vi "Run Test Suite.vi"() -> ()   [LabVIEW 2013]
uses:
  <vilib>/addons/_JKI Toolkits/Caraya/classes/Test/Test.lvclass
panel:
  out "error out":errorcluster
  # "Run Me"
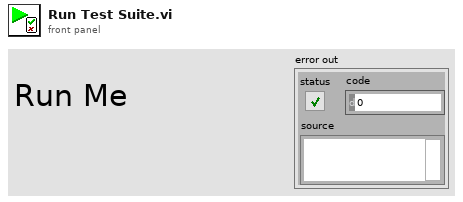
[diagram p1: front panel]
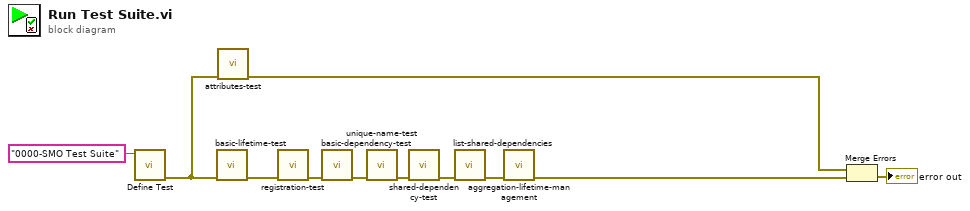
[diagram p0: block diagram]
diagram:
  n1 = call <vilib>:"Define Test.vi"("Label (VI Title)"="0000-SMO Test Suite") -> ("error out"=w1:errorcluster)  [unwired: 10 in]
  n2 = call "basic-lifetime-test.vi"("error in (no error)"=w1) -> ("error out"=w9:errorcluster)  [unwired: 10 in]
  n3 = call "attributes-test.vi"("error in (no error)"=w1) -> ("error out"=w2:errorcluster)  [unwired: 10 in]
  n4 = call "registration-test.vi"("error in (no error)"=w9) -> ("error out"=w8:errorcluster)  [unwired: 10 in]
  n5 = call "basic-dependency-test.vi"("error in (no error)"=w8) -> ("error out"=w10:errorcluster)  [unwired: 10 in]
  n6 = call "unique-name-test.vi"("error in (no error)"=w10) -> ("error out"=w7:errorcluster)  [unwired: 10 in]
  n7 = call "shared-dependency-test.vi"("error in (no error)"=w7) -> ("error out"=w6:errorcluster)  [unwired: 10 in]
  n8 = call "list-shared-dependencies.vi"("error in (no error)"=w6) -> ("error out"=w5:errorcluster)  [unwired: 10 in]
  n9 = call "aggregation-lifetime-management.vi"("error in (no error)"=w5) -> ("error out"=w4:errorcluster)  [unwired: 10 in]
  n10 = Merge Errors(w2, w4) -> (→"error out":errorcluster)
